vi "Stop Transfer Area.vi"(0 "Device ID":T1(ring), 11 "error in":errorcluster) -> (4 "Device ID Out":T1(ring), 15 "error out":errorcluster)   [LabVIEW 2010]
doc: "This VI stops the transfer area which is where the Robo Interface writes data to be read and reads data to be written."
uses:
  Robo Interface.dll
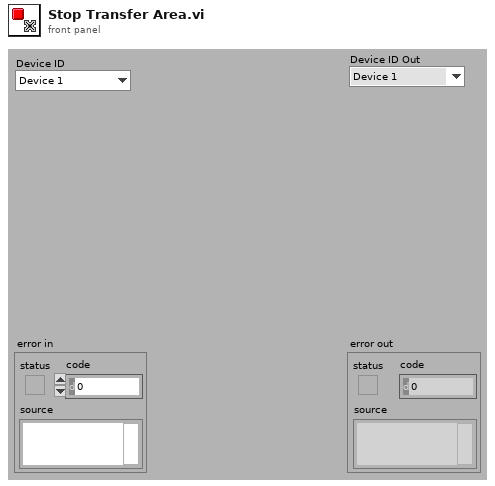
[diagram p1: front panel]
types:
  T1 = enum16{"Device 1", "Device 2", "Device 3", "Device 4", "Device 5", "Device 6", "Device 7", "Device 8"}
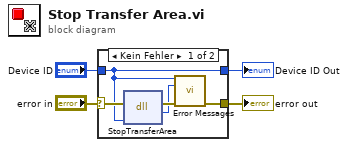
[diagram p0: block diagram]
diagram:
  n1 = case shown="Kein Fehler" "error in" {
    selector: "error in" -> [w8 w11]
    tunnel: [w7 w11] -> w1
    tunnel: "Device ID" -> [w5 w10]
    tunnel: [w5 w10] -> w2
    frame No Error {
      n2 = dll-call lib="D:/Aron/LabVIEW-Programmierung/a.F.b.u.s.A/robo_interface_distribute/Robo Interface/Advanced/Robo Interface.dll" fn="StopTransferArea"(error in=w8, "Device_ID"=w5) -> (error out=w9:errorcluster, "return type"=w6:i32)  [unwired: 2 in, 2 out]
      n3 = call "Error Messages.vi"("Device ID"=w5, "Error Code"=w6, "error in (no error)"=w9) -> ("error out"=w7:errorcluster)  [unwired: 12 out]
    }
    frame Error {
    }
  }
  "error out" <- w1
  "Device ID Out" <- w2
